vi "canDataSort.vi"() -> ()   [LabVIEW 2023] (continued)
1072  1FFFFFFF   00000004    8        00\t20\tFF\tFF\tFF\tFF\tFF\tFF\r\n      1063  0CF102A7   00000004    8        30\t75\tE0\t2E\t80\tFF\tFF\tFD\r\n      1063  0CF101A7   00000004    8        68\t00\t97\tCC\t00\t15\t39\t4F\r\n      1062  1FFFFFFF   00000004    8        00\t20\tFF\tFF\tFF\tFF\tFF\tFF\r\n      1052  1FFFFFFF   00000004    8        00\t00\tFF\tFF\tFF\tFF\tFF\tFF\r\n      1047  1FFFFFFF   00000004    8        00\t00\tFF\tFF\tFF\tFF\tFF\tFF\r\n      1046  18F121F0   00000004    8        09\t18\t00\t00\tFF\tFF\tB0\t01\r\n      1045  18F106A7   00000004    8        00\tF7\tFF\tFF\tFF\tFF\tFF\t85\r\n      1045  0CF104A7   00000004    8        F0\t60\t22\tFC\tFF\tFF\tFF\t42\r\n      1044  0CF103A7   00000004    8        17\t1F\t08\t60\tB1\t1F\t08\t42\r\n      1044  0CF102A7   00000004    8        30\t75\tE0\t2E\t80\tFF\tFF\tFD\r\n      1082  1FFFFFFF   00000004    8        00\t20\tFF\tFF\tFF\tFF\tFF\tFF\r\n      1072  1FFFFFFF   00000004    8        00\t20\tFF\tFF\tFF\tFF\tFF\tFF\r\n      1063  0CF102A7   00000004    8        30\t75\tE0\t2E\t80\tFF\tFF\tFD\r\n      1063  0CF101A7   00000004    8        68\t00\t97\tCC\t00\t15\t39\t4F\r\n      1062  1FFFFFFF   00000004    8        00\t20\tFF\tFF\tFF\tFF\tFF\tFF\r\n      1052  1FFFFFFF   00000004    8        00\t00\tFF\tFF\tFF\tFF\tFF\tFF\r\n      1047  1FFFFFFF   00000004    8        00\t00\tFF\tFF\tFF\tFF\tFF\tFF\r\n      1046  18F121F0   00000004    8        09\t18\t00\t00\tFF\tFF\tB0\t01\r\n      1045  18F106A7   00000004    8        00\tF7\tFF\tFF\tFF\tFF\tFF\t85\r\n      1045  0CF104A7   00000004    8        F0\t60\t22\tFC\tFF\tFF\tFF\t42\r\n      1044  0CF103A7   00000004    8        17\t1F\t08\t60\tB1\t1F\t08\t42\r\n      1083  0CF101A7   00000004    8        68\t00\t97\tCC\t00\t15\t39\t50\r\n      1082  1FFFFFFF   00000004    8        00\t20\tFF\tFF\tFF\tFF\tFF\tFF\r\n      1072  1FFFFFFF   00000004    8        00\t20\tFF\tFF\tFF\tFF\tFF\tFF\r\n      1063  0CF102A7   00000004    8        30\t75\tE0\t2E\t80\tFF\tFF\tFD\r\n      1063  0CF101A7   00000004    8        68\t00\t97\tCC\t00\t15\t39\t4F\r\n      1062  1FFFFFFF   00000004    8        00\t20\tFF\tFF\tFF\tFF\tFF\tFF\r\n      1052  1FFFFFFF   00000004    8        00\t00\tFF\tFF\tFF\tFF\tFF\tFF\r\n      1047  1FFFFFFF   00000004    8        00\t00\tFF\tFF\tFF\tFF\tFF\tFF\r\n      1046  18F121F0   00000004    8        09\t18\t00\t00\tFF\tFF\tB0\t01\r\n      1045  18F106A7   00000004    8        00\tF7\tFF\tFF\tFF\tFF\tFF\t85\r\n      1045  0CF104A7   00000004    8        F0\t60\t22\tFC\tFF\tFF\tFF\t42\r\n      1083  0CF102A7   00000004    8        30\t75\tE0\t2E\t80\tFF\tFF\tFD\r\n      1083  0CF101A7   00000004    8        68\t00\t97\tCC\t00\t15\t39\t50\r\n      1082  1FFFFFFF   00000004    8        00\t20\tFF\tFF\tFF\tFF\tFF\tFF\r\n      1072  1FFFFFFF   00000004    8        00\t20\tFF\tFF\tFF\tFF\tFF\tFF\r\n      1063  0CF102A7   00000004    8        30\t75\tE0\t2E\t80\tFF\tFF\tFD\r\n      1063  0CF101A7   00000004    8        68\t00\t97\tCC\t00\t15\t39\t4F\r\n      1062  1FFFFFFF   00000004    8        00\t20\tFF\tFF\tFF\tFF\tFF\tFF\r\n      1052  1FFFFFFF   00000004    8        00\t00\tFF\tFF\tFF\tFF\tFF\tFF\r\n      1047  1FFFFFFF   00000004    8        00\t00\tFF\tFF\tFF\tFF\tFF\tFF\r\n      1046  18F121F0   00000004    8        09\t18\t00\t00\tFF\tFF\tB0\t01\r\n      1045  18F106A7   00000004    8        00\tF7\tFF\tFF\tFF\tFF\tFF\t85\r\n      1092  1FFFFFFF   00000004    8        00\t00\tFF\tFF\tFF\tFF\tFF\tFF\r\n      1083  0CF102A7   00000004    8        30\t75\tE0\t2E\t80\tFF\tFF\tFD\r\n      1083  0CF101A7   00000004    8        68\t00\t97\tCC\t00\t15\t39\t50\r\n      1082  1FFFFFFF   00000004    8        00\t20\tFF\tFF\tFF\tFF\tFF\tFF\r\n      1072  1FFFFFFF   00000004    8        00\t20\tFF\tFF\tFF\tFF\tFF\tFF\r\n      1063  0CF102A7   00000004    8        30\t75\tE0\t2E\t80\tFF\tFF\tFD\r\n      1063  0CF101A7   00000004    8        68\t00\t97\tCC\t00\t15\t39\t4F\r\n      1062  1FFFFFFF   00000004    8        00\t20\tFF\tFF\tFF\tFF\tFF\tFF\r\n      1052  1FFFFFFF   00000004    8        00\t00\tFF\tFF\tFF\tFF\tFF\tFF\r\n      1047  1FFFFFFF   00000004    8        00\t00\tFF\tFF\tFF\tFF\tFF\tFF\r\n      1046  18F121F0   00000004    8        09\t18\t00\t00\tFF\tFF\tB0\t01\r\n      1093  18F106A7   00000004    8        00\tF7\tFF\tFF\tFF\tFF\tFF\t86\r\n      1092  1FFFFFFF   00000004    8        00\t00\tFF\tFF\tFF\tFF\tFF\tFF\r\n      1083  0CF102A7   00000004    8        30\t75\tE0\t2E\t80\tFF\tFF\tFD\r\n      1083  0CF101A7   00000004    8        68\t00\t97\tCC\t00\t15\t39\t50\r\n      1082  1FFFFFFF   00000004    8        00\t20\tFF\tFF\tFF\tFF\tFF\tFF\r\n      1072  1FFFFFFF   00000004    8        00\t20\tFF\tFF\tFF\tFF\tFF\tFF\r\n      1063  0CF102A7   00000004    8        30\t75\tE0\t2E\t80\tFF\tFF\tFD\r\n      1063  0CF101A7   00000004    8        68\t00\t97\tCC\t00\t15\t39\t4F\r\n      1062  1FFFFFFF   00000004    8        00\t20\tFF\tFF\tFF\tFF\tFF\tFF\r\n      1052  1FFFFFFF   00000004    8        00\t00\tFF\tFF\tFF\tFF\tFF\tFF\r\n      1047  1FFFFFFF   00000004    8        00\t00\tFF\tFF\tFF\tFF\tFF\tFF\r\n      1102  1FFFFFFF   00000004    8        00\t20\tFF\tFF\tFF\tFF\tFF\tFF\r\n      1093  18F106A7   00000004    8        00\tF7\tFF\tFF\tFF\tFF\tFF\t86\r\n      1092  1FFFFFFF   00000004    8        00\t00\tFF\tFF\tFF\tFF\tFF\tFF\r\n      1083  0CF102A7   00000004    8        30\t75\tE0\t2E\t80\tFF\tFF\tFD\r\n      1083  0CF101A7   00000004    8        68\t00\t97\tCC\t00\t15\t39\t50\r\n      1082  1FFFFFFF   00000004    8        00\t20\tFF\tFF\tFF\tFF\tFF\tFF\r\n      1072  1FFFFFFF   00000004    8        00\t20\tFF\tFF\tFF\tFF\tFF\tFF\r\n      1063  0CF102A7   00000004    8        30\t75\tE0\t2E\t80\tFF\tFF\tFD\r\n      1063  0CF101A7   00000004    8        68\t00\t97\tCC\t00\t15\t39\t4F\r\n      1062  1FFFFFFF   00000004    8        00\t20\tFF\tFF\tFF\tFF\tFF\tFF\r\n      1052  1FFFFFFF   00000004    8        00\t00\tFF\tFF\tFF\tFF\tFF\tFF\r\n      1103  0CF101A7   00000004    8        68\t00\t97\tCC\t00\t15\t39\t51\r\n      1102  1FFFFFFF   00000004    8        00\t20\tFF\tFF\tFF\tFF\tFF\tFF\r\n      1093  18F106A7   00000004    8        00\tF7\tFF\tFF\tFF\tFF\tFF\t86\r\n      1092  1FFFFFFF   00000004    8        00\t00\tFF\tFF\tFF\tFF\tFF\tFF\r\n      1083  0CF102A7   00000004    8        30\t75\tE0\t2E\t80\tFF\tFF\tFD\r\n      1083  0CF101A7   00000004    8        68\t00\t97\tCC\t00\t15\t39\t50\r\n      1082  1FFFFFFF   00000004    8        00\t20\tFF\tFF\tFF\tFF\tFF\tFF\r\n      1072  1FFFFFFF   00000004    8        00\t20\tFF\tFF\tFF\tFF\tFF\tFF\r\n      1063  0CF102A7   00000004    8        30\t75\tE0\t2E\t80\tFF\tFF\tFD\r\n      1063  0CF101A7   00000004    8        68\t00\t97\tCC\t00\t15\t39\t4F\r\n      1062  1FFFFFFF   00000004    8        00\t20\tFF\tFF\tFF\tFF\tFF\tFF\r\n      1103  0CF102A7   00000004    8        30\t75\tE0\t2E\t80\tFF\tFF\tFD\r\n      1103  0CF101A7   00000004    8        68\t00\t97\tCC\t00\t15\t39\t51\r\n      1102  1FFFFFFF   00000004    8        00\t20\tFF\tFF\tFF\tFF\tFF\tFF\r\n      1093  18F106A7   00000004    8        00\tF7\tFF\tFF\tFF\tFF\tFF\t86\r\n      1092  1FFFFFFF   00000004    8        00\t00\tFF\tFF\tFF\tFF\tFF\tFF\r\n      1083  0CF102A7   00000004    8        30\t75\tE0\t2E\t80\tFF\tFF\tFD\r\n      1083  0CF101A7   00000004    8        68\t00\t97\tCC\t00\t15\t39\t50\r\n      1082  1FFFFFFF   00000004    8        00\t20\tFF\tFF\tFF\tFF\tFF\tFF\r\n      1072  1FFFFFFF   00000004    8        00\t20\tFF\tFF\tFF\tFF\tFF\tFF\r\n      1063  0CF102A7   00000004    8        30\t75\tE0\t2E\t80\tFF\tFF\tFD\r\n      1063  0CF101A7   00000004    8        68\t00\t97\tCC\t00\t15\t39\t4F\r\n      1112  1FFFFFFF   00000004    8        00\t20\tFF\tFF\tFF\tFF\tFF\tFF\r\n      1103  0CF102A7   00000004    8        30\t75\tE0\t2E\t80\tFF\tFF\tFD\r\n      1103  0CF101A7   00000004    8        68\t00\t97\tCC\t00\t15\t39\t51\r\n      1102  1FFFFFFF   00000004    8        00\t20\tFF\tFF\tFF\tFF\tFF\tFF\r\n      1093  18F106A7   00000004    8        00\tF7\tFF\tFF\tFF\tFF\tFF\t86\r\n      1092  1FFFFFFF   00000004    8        00\t00\tFF\tFF\tFF\tFF\tFF\tFF\r\n      1083  0CF102A7   00000004    8        30\t75\tE0\t2E\t80\tFF\tFF\tFD\r\n      1083  0CF101A7   00000004    8        68\t00\t97\tCC\t00\t15\t39\t50\r\n      1082  1FFFFFFF   00000004    8        00\t20\tFF\tFF\tFF\tFF\tFF\tFF\r\n      1072  1FFFFFFF   00000004    8        00\t20\tFF\tFF\tFF\tFF\tFF\tFF\r\n      1063  0CF102A7   00000004    8        30\t75\tE0\t2E\t80\tFF\tFF\tFD\r\n      1122  1FFFFFFF   00000004    8        00\t20\tFF\tFF\tFF\tFF\tFF\tFF\r\n      1112  1FFFFFFF   00000004    8        00\t20\tFF\tFF\tFF\tFF\tFF\tFF\r\n      1103  0CF102A7   00000004    8        30\t75\tE0\t2E\t80\tFF\tFF\tFD\r\n      1103  0CF101A7   00000004    8        68\t00\t97\tCC\t00\t15\t39\t51\r\n      1102  1FFFFFFF   00000004    8        00\t20\tFF\tFF\tFF\tFF\tFF\tFF\r\n      1093  18F106A7   00000004    8        00\tF7\tFF\tFF\tFF\tFF\tFF\t86\r\n      1092  1FFFFFFF   00000004    8        00\t00\tFF\tFF\tFF\tFF\tFF\tFF\r\n      1083  0CF102A7   00000004    8        30\t75\tE0\t2E\t80\tFF\tFF\tFD\r\n      1083  0CF101A7   00000004    8        68\t00\t97\tCC\t00\t15\t39\t50\r\n      1082  1FFFFFFF   00000004    8        00\t20\tFF\tFF\tFF\tFF\tFF\tFF\r\n      1072  1FFFFFFF   00000004    8        00\t20\tFF\tFF\tFF\tFF\tFF\tFF\r\n      1123  0CF101A7   00000004    8        68\t00\t97\tCC\t00\t15\t39\t52\r\n      1122  1FFFFFFF   00000004    8        00\t20\tFF\tFF\tFF\tFF\tFF\tFF\r\n      1112  1FFFFFFF   00000004    8        00\t20\tFF\tFF\tFF\tFF\tFF\tFF\r\n      1103  0CF102A7   00000004    8        30\t75\tE0\t2E\t80\tFF\tFF\tFD\r\n      1103  0CF101A7   00000004    8        68\t00\t97\tCC\t00\t15\t39\t51\r\n      1102  1FFFFFFF   00000004    8        00\t20\tFF\tFF\tFF\tFF\tFF\tFF\r\n      1093  18F106A7   00000004    8        00\tF7\tFF\tFF\tFF\tFF\tFF\t86\r\n      1092  1FFFFFFF   00000004    8        00\t00\tFF\tFF\tFF\tFF\tFF\tFF\r\n      1083  0CF102A7   00000004    8        30\t75\tE0\t2E\t80\tFF\tFF\tFD\r\n      1083  0CF101A7   00000004    8        68\t00\t97\tCC\t00\t15\t39\t50\r\n      1082  1FFFFFFF   00000004    8        00\t20\tFF\tFF\tFF\tFF\tFF\tFF\r\n      1123  0CF102A7   00000004    8        30\t75\tE0\t2E\t80\tFF\tFF\tFD\r\n      1123  0CF101A7   00000004    8        68\t00\t97\tCC\t00\t15\t39\t52\r\n      1122  1FFFFFFF   00000004    8        00\t20\tFF\tFF\tFF\tFF\tFF\tFF\r\n      1112  1FFFFFFF   00000004    8        00\t20\tFF\tFF\tFF\tFF\tFF\tFF\r\n      1103  0CF102A7   00000004    8        30\t75\tE0\t2E\t80\tFF\tFF\tFD\r\n      1103  0CF101A7   00000004    8        68\t00\t97\tCC\t00\t15\t39\t51\r\n      1102  1FFFFFFF   00000004    8        00\t20\tFF\tFF\tFF\tFF\tFF\tFF\r\n      1093  18F106A7   00000004    8        00\tF7\tFF\tFF\tFF\tFF\tFF\t86\r\n      1092  1FFFFFFF   00000004    8        00\t00\tFF\tFF\tFF\tFF\tFF\tFF\r\n      1083  0CF102A7   00000004    8        30\t75\tE0\t2E\t80\tFF\tFF\tFD\r\n      1083  0CF101A7   00000004    8        68\t00\t97\tCC\t00\t15\t39\t50\r\n      1132  1FFFFFFF   00000004    8        00\t20\tFF\tFF\tFF\tFF\tFF\tFF\r\n      1123  0CF102A7   00000004    8        30\t75\tE0\t2E\t80\tFF\tFF\tFD\r\n      1123  0CF101A7   00000004    8        68\t00\t97\tCC\t00\t15\t39\t52\r\n      1122  1FFFFFFF   00000004    8        00\t20\tFF\tFF\tFF\tFF\tFF\tFF\r\n      1112  1FFFFFFF   00000004    8        00\t20\tFF\tFF\tFF\tFF\tFF\tFF\r\n      1103  0CF102A7   00000004    8        30\t75\tE0\t2E\t80\tFF\tFF\tFD\r\n      1103  0CF101A7   00000004    8        68\t00\t97\tCC\t00\t15\t39\t51\r\n      1102  1FFFFFFF   00000004    8        00\t20\tFF\tFF\tFF\tFF\tFF\tFF\r\n      1093  18F106A7   00000004    8        00\tF7\tFF\tFF\tFF\tFF\tFF\t86\r\n      1092  1FFFFFFF   00000004    8        00\t00\tFF\tFF\tFF\tFF\tFF\tFF\r\n      1083  0CF102A7   00000004    8        30\t75\tE0\t2E\t80\tFF\tFF\tFD\r\n      1141  18F11FF0   00000004    8        FF\t3F\t90\t68\t88\t1B\t10\t3C\r\n      1132  1FFFFFFF   00000004    8        00\t20\tFF\tFF\tFF\tFF\tFF\tFF\r\n      1123  0CF102A7   00000004    8        30\t75\tE0\t2E\t80\tFF\tFF\tFD\r\n      1123  0CF101A7   00000004    8        68\t00\t97\tCC\t00\t15\t39\t52\r\n      1122  1FFFFFFF   00000004    8        00\t20\tFF\tFF\tFF\tFF\tFF\tFF\r\n      1112  1FFFFFFF   00000004    8        00\t20\tFF\tFF\tFF\tFF\tFF\tFF\r\n      1103  0CF102A7   00000004    8        30\t75\tE0\t2E\t80\tFF\tFF\tFD\r\n      1103  0CF101A7   00000004    8        68\t00\t97\tCC\t00\t15\t39\t51\r\n      1102  1FFFFFFF   00000004    8        00\t20\tFF\tFF\tFF\tFF\tFF\tFF\r\n      1093  18F106A7   00000004    8        00\tF7\tFF\tFF\tFF\tFF\tFF\t86\r\n      1092  1FFFFFFF   00000004    8        00\t00\tFF\tFF\tFF\tFF\tFF\tFF\r\n      1142  18F120F0   00000004    8        2B\t75\t60\tB1\tB0\t01\tFF\tFF\r\n      1141  18F11FF0   00000004    8        FF\t3F\t90\t68\t88\t1B\t10\t3C\r\n      1132  1FFFFFFF   00000004    8        00\t20\tFF\tFF\tFF\tFF\tFF\tFF\r\n      1123  0CF102A7   00000004    8        30\t75\tE0\t2E\t80\tFF\tFF\tFD\r\n      1123  0CF101A7   00000004    8        68\t00\t97\tCC\t00\t15\t39\t52\r\n      1122  1FFFFFFF   00000004    8        00\t20\tFF\tFF\tFF\tFF\tFF\tFF\r\n      1112  1FFFFFFF   00000004    8        00\t20\tFF\tFF\tFF\tFF\tFF\tFF\r\n      1103  0CF102A7   00000004    8        30\t75\tE0\t2E\t80\tFF\tFF\tFD\r\n      1103  0CF101A7   00000004    8        68\t00\t97\tCC\t00\t15\t39\t51\r\n      1102  1FFFFFFF   00000004    8        00\t20\tFF\tFF\tFF\tFF\tFF\tFF\r\n      1093  18F106A7   00000004    8        00\tF7\tFF\tFF\tFF\tFF\tFF\t86\r\n      1143  0CF101A7   00000004    8        68\t00\t97\tCC\t00\t15\t39\t53\r\n      1142  18F120F0   00000004    8        2B\t75\t60\tB1\tB0\t01\tFF\tFF\r\n      1141  18F11FF0   00000004    8        FF\t3F\t90\t68\t88\t1B\t10\t3C\r\n      1132  1FFFFFFF   00000004    8        00\t20\tFF\tFF\tFF\tFF\tFF\tFF\r\n      1123  0CF102A7   00000004    8        30\t75\tE0\t2E\t80\tFF\tFF\tFD\r\n      1123  0CF101A7   00000004    8        68\t00\t97\tCC\t00\t15\t39\t52\r\n      1122  1FFFFFFF   00000004    8        00\t20\tFF\tFF\tFF\tFF\tFF\tFF\r\n      1112  1FFFFFFF   00000004    8        00\t20\tFF\tFF\tFF\tFF\tFF\tFF\r\n      1103  0CF102A7   00000004    8        30\t75\tE0\t2E\t80\tFF\tFF\tFD\r\n      1103  0CF101A7   00000004    8        68\t00\t97\tCC\t00\t15\t39\t51\r\n      1102  1FFFFFFF   00000004    8        00\t20\tFF\tFF\tFF\tFF\tFF\tFF\r\n      1143  0C3C4D4A   00000004    8        BE\tFF\tFF\t7F\t18\tFF\tFF\t43\r\n      1143  0CF101A7   00000004    8        68\t00\t97\tCC\t00\t15\t39\t53\r\n      1142  18F120F0   00000004    8        2B\t75\t60\tB1\tB0\t01\tFF\tFF\r\n      1141  18F11FF0   00000004    8        FF\t3F\t90\t68\t88\t1B\t10\t3C\r\n      1132  1FFFFFFF   00000004    8        00\t20\tFF\tFF\tFF\tFF\tFF\tFF\r\n      1123  0CF102A7   00000004    8        30\t75\tE0\t2E\t80\tFF\tFF\tFD\r\n      1123  0CF101A7   00000004    8        68\t00\t97\tCC\t00\t15\t39\t52\r\n      1122  1FFFFFFF   00000004    8        00\t20\tFF\tFF\tFF\tFF\tFF\tFF\r\n      1112  1FFFFFFF   00000004    8        00\t20\tFF\tFF\tFF\tFF\tFF\tFF\r\n      1103  0CF102A7   00000004    8        30\t75\tE0\t2E\t80\tFF\tFF\tFD\r\n      1103  0CF101A7   00000004    8        68\t00\t97\tCC\t00\t15\t39\t51\r\n      1144  0CF102A7   00000004    8        30\t75\tE0\t2E\t80\tFF\tFF\tFD\r\n      1143  0C3C4D4A   00000004    8        BE\tFF\tFF\t7F\t18\tFF\tFF\t43\r\n      1143  0CF101A7   00000004    8        68\t00\t97\tCC\t00\t15\t39\t53\r\n      1142  18F120F0   00000004    8        2B\t75\t60\tB1\tB0\t01\tFF\tFF\r\n      1141  18F11FF0   00000004    8        FF\t3F\t90\t68\t88\t1B\t10\t3C\r\n      1132  1FFFFFFF   00000004    8        00\t20\tFF\tFF\tFF\tFF\tFF\tFF\r\n      1123  0CF102A7   00000004    8        30\t75\tE0\t2E\t80\tFF\tFF\tFD\r\n      1123  0CF101A7   00000004    8        68\t00\t97\tCC\t00\t15\t39\t52\r\n      1122  1FFFFFFF   00000004    8        00\t20\tFF\tFF\tFF\tFF\tFF\tFF\r\n      1112  1FFFFFFF   00000004    8        00\t20\tFF\tFF\tFF\tFF\tFF\tFF\r\n      1103  0CF102A7   00000004    8        30\t75\tE0\t2E\t80\tFF\tFF\tFD\r\n      1144  0CF103A7   00000004    8        17\t1F\t08\t60\tB1\t1F\t08\t43\r\n      1144  0CF102A7   00000004    8        30\t75\tE0\t2E\t80\tFF\tFF\tFD\r\n      1143  0C3C4D4A   00000004    8        BE\tFF\tFF\t7F\t18\tFF\tFF\t43\r\n      1143  0CF101A7   00000004    8        68\t00\t97\tCC\t00\t15\t39\t53\r\n      1142  18F120F0   00000004    8        2B\t75\t60\tB1\tB0\t01\tFF\tFF\r\n      1141  18F11FF0   00000004    8        FF\t3F\t90\t68\t88\t1B\t10\t3C\r\n      1132  1FFFFFFF   00000004    8        00\t20\tFF\tFF\tFF\tFF\tFF\tFF\r\n      1123  0CF102A7   00000004    8        30\t75\tE0\t2E\t80\tFF\tFF\tFD\r\n      1123  0CF101A7   00000004    8        68\t00\t97\tCC\t00\t15\t39\t52\r\n      1122  1FFFFFFF   00000004    8        00\t20\tFF\tFF\tFF\tFF\tFF\tFF\r\n      1112  1FFFFFFF   00000004    8        00\t20\tFF\tFF\tFF\tFF\tFF\tFF\r\n      1145  0CF104A7   00000004    8        F0\t60\t22\tFC\tFF\tFF\tFF\t43\r\n      1144  0CF103A7   00000004    8        17\t1F\t08\t60\tB1\t1F\t08\t43\r\n      1144  0CF102A7   00000004    8        30\t75\tE0\t2E\t80\tFF\tFF\tFD\r\n      1143  0C3C4D4A   00000004    8        BE\tFF\tFF\t7F\t18\tFF\tFF\t43\r\n      1143  0CF101A7   00000004    8        68\t00\t97\tCC\t00\t15\t39\t53\r\n      1142  18F120F0   00000004    8        2B\t75\t60\tB1\tB0\t01\tFF\tFF\r\n      1141  18F11FF0   00000004    8        FF\t3F\t90\t68\t88\t1B\t10\t3C\r\n      1132  1FFFFFFF   00000004    8        00\t20\tFF\tFF\tFF\tFF\tFF\tFF\r\n      1123  0CF102A7   00000004    8        30\t75\tE0\t2E\t80\tFF\tFF\tFD\r\n      1123  0CF101A7   00000004    8        68\t00\t97\tCC\t00\t15\t39\t52\r\n      1122  1FFFFFFF   00000004    8        00\t20\tFF\tFF\tFF\tFF\tFF\tFF\r\n      1145  18F106A7   00000004    8        00\tF7\tFF\tFF\tFF\tFF\tFF\t87\r\n      1145  0CF104A7   00000004    8        F0\t60\t22\tFC\tFF\tFF\tFF\t43\r\n      1144  0CF103A7   00000004    8        17\t1F\t08\t60\tB1\t1F\t08\t43\r\n      1144  0CF102A7   00000004    8        30\t75\tE0\t2E\t80\tFF\tFF\tFD\r\n      1143  0C3C4D4A   00000004    8        BE\tFF\tFF\t7F\t18\tFF\tFF\t43\r\n      1143  0CF101A7   00000004    8        68\t00\t97\tCC\t00\t15\t39\t53\r\n      1142  18F120F0   00000004    8        2B\t75\t60\tB1\tB0\t01\tFF\tFF\r\n      1141  18F11FF0   00000004    8        FF\t3F\t90\t68\t88\t1B\t10\t3C\r\n      1132  1FFFFFFF   00000004    8        00\t20\tFF\tFF\tFF\tFF\tFF\tFF\r\n      1123  0CF102A7   00000004    8        30\t75\tE0\t2E\t80\tFF\tFF\tFD\r\n      1123  0CF101A7   00000004    8        68\t00\t97\tCC\t00\t15\t39\t52\r\n      1146  18F108A7   00000004    8        F0\t00\t00\tFF\tFF\tFF\tFF\t40\r\n      1145  18F106A7   00000004    8        00\tF7\tFF\tFF\tFF\tFF\tFF\t87\r\n      1145  0CF104A7   00000004    8        F0\t60\t22\tFC\tFF\tFF\tFF\t43\r\n      1144  0CF103A7   00000004    8        17\t1F\t08\t60\tB1\t1F\t08\t43\r\n      1144  0CF102A7   00000004    8        30\t75\tE0\t2E\t80\tFF\tFF\tFD\r\n      1143  0C3C4D4A   00000004    8        BE\tFF\tFF\t7F\t18\tFF\tFF\t43\r\n      1143  0CF101A7   00000004    8        68\t00\t97\tCC\t00\t15\t39\t53\r\n      1142  18F120F0   00000004    8        2B\t75\t60\tB1\tB0\t01\tFF\tFF\r\n      1141  18F11FF0   00000004    8        FF\t3F\t90\t68\t88\t1B\t10\t3C\r\n      1132  1FFFFFFF   00000004    8        00\t20\tFF\tFF\tFF\tFF\tFF\tFF\r\n      1123  0CF102A7   00000004    8        30\t75\tE0\t2E\t80\tFF\tFF\tFD\r\n      1147  18F121F0   00000004    8        09\t18\t00\t00\tFF\tFF\tB0\t01\r\n      1146  18F108A7   00000004    8        F0\t00\t00\tFF\tFF\tFF\tFF\t40\r\n      1145  18F106A7   00000004    8        00\tF7\tFF\tFF\tFF\tFF\tFF\t87\r\n      1145  0CF104A7   00000004    8        F0\t60\t22\tFC\tFF\tFF\tFF\t43\r\n      1144  0CF103A7   00000004    8        17\t1F\t08\t60\tB1\t1F\t08\t43\r\n      1144  0CF102A7   00000004    8        30\t75\tE0\t2E\t80\tFF\tFF\tFD\r\n      1143  0C3C4D4A   00000004    8        BE\tFF\tFF\t7F\t18\tFF\tFF\t43\r\n      1143  0CF101A7   00000004    8        68\t00\t97\tCC\t00\t15\t39\t53\r\n      1142  18F120F0   00000004    8        2B\t75\t60\tB1\tB0\t01\tFF\tFF\r\n      1141  18F11FF0   00000004    8        FF\t3F\t90\t68\t88\t1B\t10\t3C\r\n      1132  1FFFFFFF   00000004    8        00\t20\tFF\tFF\tFF\tFF\tFF\tFF\r\n      1147  18FEF117   00000004    8        F7\t97\tCC\tCF\tFF\tFF\tFF\tFF\r\n      1147  18F121F0   00000004    8        09\t18\t00\t00\tFF\tFF\tB0\t01\r\n      1146  18F108A7   00000004    8        F0\t00\t00\tFF\tFF\tFF\tFF\t40\r\n      1145  18F106A7   00000004    8        00\tF7\tFF\tFF\tFF\tFF\tFF\t87\r\n      1145  0CF104A7   00000004    8        F0\t60\t22\tFC\tFF\tFF\tFF\t43\r\n      1144  0CF103A7   00000004    8        17\t1F\t08\t60\tB1\t1F\t08\t43\r\n      1144  0CF102A7   00000004    8        30\t75\tE0\t2E\t80\tFF\tFF\tFD\r\n      1143  0C3C4D4A   00000004    8        BE\tFF\tFF\t7F\t18\tFF\tFF\t43\r\n      1143  0CF101A7   00000004    8        68\t00\t97\tCC\t00\t15\t39\t53\r\n      1142  18F120F0   00000004    8        2B\t75\t60\tB1\tB0\t01\tFF\tFF\r\n      1141  18F11FF0   00000004    8        FF\t3F\t90\t68\t88\t1B\t10\t3C\r\n      1148  1FFFFFFF   00000004    8        00\t00\tFF\tFF\tFF\tFF\tFF\tFF\r\n      1147  18FEF117   00000004    8        F7\t97\tCC\tCF\tFF\tFF\tFF\tFF\r\n      1147  18F121F0   00000004    8        09\t18\t00\t00\tFF\tFF\tB0\t01\r\n      1146  18F108A7   00000004    8        F0\t00\t00\tFF\tFF\tFF\tFF\t40\r\n      1145  18F106A7   00000004    8        00\tF7\tFF\tFF\tFF\tFF\tFF\t87\r\n      1145  0CF104A7   00000004    8        F0\t60\t22\tFC\tFF\tFF\tFF\t43\r\n      1144  0CF103A7   00000004    8        17\t1F\t08\t60\tB1\t1F\t08\t43\r\n      1144  0CF102A7   00000004    8        30\t75\tE0\t2E\t80\tFF\tFF\tFD\r\n      1143  0C3C4D4A   00000004    8        BE\tFF\tFF\t7F\t18\tFF\tFF\t43\r\n      1143  0CF101A7   00000004    8        68\t00\t97\tCC\t00\t15\t39\t53\r\n      1142  18F120F0   00000004    8        2B\t75\t60\tB1\tB0\t01\tFF\tFF\r\n      1152  1FFFFFFF   00000004    8        00\t20\tFF\tFF\tFF\tFF\tFF\tFF\r\n      1148  1FFFFFFF   00000004    8        00\t00\tFF\tFF\tFF\tFF\tFF\tFF\r\n      1147  18FEF117   00000004    8        F7\t97\tCC\tCF\tFF\tFF\tFF\tFF\r\n      1147  18F121F0   00000004    8        09\t18\t00\t00\tFF\tFF\tB0\t01\r\n      1146  18F108A7   00000004    8        F0\t00\t00\tFF\tFF\tFF\tFF\t40\r\n      1145  18F106A7   00000004    8        00\tF7\tFF\tFF\tFF\tFF\tFF\t87\r\n      1145  0CF104A7   00000004    8        F0\t60\t22\tFC\tFF\tFF\tFF\t43\r\n      1144  0CF103A7   00000004    8        17\t1F\t08\t60\tB1\t1F\t08\t43\r\n      1144  0CF102A7   00000004    8        30\t75\tE0\t2E\t80\tFF\tFF\tFD\r\n      1143  0C3C4D4A   00000004    8        BE\tFF\tFF\t7F\t18\tFF\tFF\t43\r\n      1143  0CF101A7   00000004    8        68\t00\t97\tCC\t00\t15\t39\t53\r\n      1162  1FFFFFFF   00000004    8        00\t20\tFF\tFF\tFF\tFF\tFF\tFF\r\n      1152  1FFFFFFF   00000004    8        00\t20\tFF\tFF\tFF\tFF\tFF\tFF\r\n      1148  1FFFFFFF   00000004    8        00\t00\tFF\tFF\tFF\tFF\tFF\tFF\r\n      1147  18FEF117   00000004    8        F7\t97\tCC\tCF\tFF\tFF\tFF\tFF\r\n      1147  18F121F0   00000004    8        09\t18\t00\t00\tFF\tFF\tB0\t01\r\n      1146  18F108A7   00000004    8        F0\t00\t00\tFF\tFF\tFF\tFF\t40\r\n      1145  18F106A7   00000004    8        00\tF7\tFF\tFF\tFF\tFF\tFF\t87\r\n      1145  0CF104A7   00000004    8        F0\t60\t22\tFC\tFF\tFF\tFF\t43\r\n      1144  0CF103A7   00000004    8        17\t1F\t08\t60\tB1\t1F\t08\t43\r\n      1144  0CF102A7   00000004    8        30\t75\tE0\t2E\t80\tFF\tFF\tFD\r\n      1143  0C3C4D4A   00000004    8        BE\tFF\tFF\t7F\t18\tFF\tFF\t43\r\n      1163  0CF101A7   00000004    8        68\t00\t97\tCC\t00\t15\t39\t54\r\n      1162  1FFFFFFF   00000004    8        00\t20\tFF\tFF\tFF\tFF\tFF\tFF\r\n      1152  1FFFFFFF   00000004    8        00\t20\tFF\tFF\tFF\tFF\tFF\tFF\r\n      1148  1FFFFFFF   00000004    8        00\t00\tFF\tFF\tFF\tFF\tFF\tFF\r\n      1147  18FEF117   00000004    8        F7\t97\tCC\tCF\tFF\tFF\tFF\tFF\r\n      1147  18F121F0   00000004    8        09\t18\t00\t00\tFF\tFF\tB0\t01\r\n      1146  18F108A7   00000004    8        F0\t00\t00\tFF\tFF\tFF\tFF\t40\r\n      1145  18F106A7   00000004    8        00\tF7\tFF\tFF\tFF\tFF\tFF\t87\r\n      1145  0CF104A7   00000004    8        F0\t60\t22\tFC\tFF\tFF\tFF\t43\r\n      1144  0CF103A7   00000004    8        17\t1F\t08\t60\tB1\t1F\t08\t43\r\n      1144  0CF102A7   00000004    8        30\t75\tE0\t2E\t80\tFF\tFF\tFD\r\n      1163  0CF102A7   00000004    8        30\t75\tE0\t2E\t80\tFF\tFF\tFD\r\n      1163  0CF101A7   00000004    8        68\t00\t97\tCC\t00\t15\t39\t54\r\n      1162  1FFFFFFF   00000004    8        00\t20\tFF\tFF\tFF\tFF\tFF\tFF\r\n      1152  1FFFFFFF   00000004    8        00\t20\tFF\tFF\tFF\tFF\tFF\tFF\r\n      1148  1FFFFFFF   00000004    8        00\t00\tFF\tFF\tFF\tFF\tFF\tFF\r\n      1147  18FEF117   00000004    8        F7\t97\tCC\tCF\tFF\tFF\tFF\tFF\r\n      1147  18F121F0   00000004    8        09\t18\t00\t00\tFF\tFF\tB0\t01\r\n      1146  18F108A7   00000004    8        F0\t00\t00\tFF\tFF\tFF\tFF\t40\r\n      1145  18F106A7   00000004    8        00\tF7\tFF\tFF\tFF\tFF\tFF\t87\r\n      1145  0CF104A7   00000004    8        F0\t60\t22\tFC\tFF\tFF\tFF\t43\r\n      1144  0CF103A7   00000004    8        17\t1F\t08\t60\tB1\t1F\t08\t43\r\n      1172  1FFFFFFF   00000004    8        00\t20\tFF\tFF\tFF\tFF\tFF\tFF\r\n      1163  0CF102A7   00000004    8        30\t75\tE0\t2E\t80\tFF\tFF\tFD\r\n      1163  0CF101A7   00000004    8        68\t00\t97\tCC\t00\t15\t39\t54\r\n      1162  1FFFFFFF   00000004    8        00\t20\tFF\tFF\tFF\tFF\tFF\tFF\r\n      1152  1FFFFFFF   00000004    8        00\t20\tFF\tFF\tFF\tFF\tFF\tFF\r\n      1148  1FFFFFFF   00000004    8        00\t00\tFF\tFF\tFF\tFF\tFF\tFF\r\n      1147  18FEF117   00000004    8        F7\t97\tCC\tCF\tFF\tFF\tFF\tFF\r\n      1147  18F121F0   00000004    8        09\t18\t00\t00\tFF\tFF\tB0\t01\r\n      1146  18F108A7   00000004    8        F0\t00\t00\tFF\tFF\tFF\tFF\t40\r\n      1145  18F106A7   00000004    8        00\tF7\tFF\tFF\tFF\tFF\tFF\t87\r\n      1145  0CF104A7   00000004    8        F0\t60\t22\tFC\tFF\tFF\tFF\t43\r\n      1182  1FFFFFFF   00000004    8        00\t00\tFF\tFF\tFF\tFF\tFF\tFF\r\n      1172  1FFFFFFF   00000004    8        00\t20\tFF\tFF\tFF\tFF\tFF\tFF\r\n      1163  0CF102A7   00000004    8        30\t75\tE0\t2E\t80\tFF\tFF\tFD\r\n      1163  0CF101A7   00000004    8        68\t00\t97\tCC\t00\t15\t39\t54\r\n      1162  1FFFFFFF   00000004    8        00\t20\tFF\tFF\tFF\tFF\tFF\tFF\r\n      1152  1FFFFFFF   00000004    8        00\t20\tFF\tFF\tFF\tFF\tFF\tFF\r\n      1148  1FFFFFFF   00000004    8        00\t00\tFF\tFF\tFF\tFF\tFF\tFF\r\n      1147  18FEF117   00000004    8        F7\t97\tCC\tCF\tFF\tFF\tFF\tFF\r\n      1147  18F121F0   00000004    8        09\t18\t00\t00\tFF\tFF\tB0\t01\r\n      1146  18F108A7   00000004    8        F0\t00\t00\tFF\tFF\tFF\tFF\t40\r\n      1145  18F106A7   00000004    8        00\tF7\tFF\tFF\tFF\tFF\tFF\t87\r\n      1183  0CF101A7   00000004    8        68\t00\t97\tCC\t00\t15\t39\t55\r\n      1182  1FFFFFFF   00000004    8        00\t00\tFF\tFF\tFF\tFF\tFF\tFF\r\n      1172  1FFFFFFF   00000004    8        00\t20\tFF\tFF\tFF\tFF\tFF\tFF\r\n      1163  0CF102A7   00000004    8        30\t75\tE0\t2E\t80\tFF\tFF\tFD\r\n      1163  0CF101A7   00000004    8        68\t00\t97\tCC\t00\t15\t39\t54\r\n      1162  1FFFFFFF   00000004    8        00\t20\tFF\tFF\tFF\tFF\tFF\tFF\r\n      1152  1FFFFFFF   00000004    8        00\t20\tFF\tFF\tFF\tFF\tFF\tFF\r\n      1148  1FFFFFFF   00000004    8        00\t00\tFF\tFF\tFF\tFF\tFF\tFF\r\n      1147  18FEF117   00000004    8        F7\t97\tCC\tCF\tFF\tFF\tFF\tFF\r\n      1147  18F121F0   00000004    8        09\t18\t00\t00\tFF\tFF\tB0\t01\r\n      1146  18F108A7   00000004    8        F0\t00\t00\tFF\tFF\tFF\tFF\t40\r\n      1183  0CF102A7   00000004    8        30\t75\tE0\t2E\t80\tFF\tFF\tFD\r\n      1183  0CF101A7   00000004    8        68\t00\t97\tCC\t00\t15\t39\t55\r\n      1182  1FFFFFFF   00000004    8        00\t00\tFF\tFF\tFF\tFF\tFF\tFF\r\n      1172  1FFFFFFF   00000004    8        00\t20\tFF\tFF\tFF\tFF\tFF\tFF\r\n      1163  0CF102A7   00000004    8        30\t75\tE0\t2E\t80\tFF\tFF\tFD\r\n      1163  0CF101A7   00000004    8        68\t00\t97\tCC\t00\t15\t39\t54\r\n      1162  1FFFFFFF   00000004    8        00\t20\tFF\tFF\tFF\tFF\tFF\tFF\r\n      1152  1FFFFFFF   00000004    8        00\t20\tFF\tFF\tFF\tFF\tFF\tFF\r\n      1148  1FFFFFFF   00000004    8        00\t00\tFF\tFF\tFF\tFF\tFF\tFF\r\n      1147  18FEF117   00000004    8        F7\t97\tCC\tCF\tFF\tFF\tFF\tFF\r\n      1147  18F121F0   00000004    8        09\t18\t00\t00\tFF\tFF\tB0\t01\r\n      1192  1FFFFFFF   00000004    8        00\t20\tFF\tFF\tFF\tFF\tFF\tFF\r\n      1183  0CF102A7   00000004    8        30\t75\tE0\t2E\t80\tFF\tFF\tFD\r\n      1183  0CF101A7   00000004    8        68\t00\t97\tCC\t00\t15\t39\t55\r\n      1182  1FFFFFFF   00000004    8        00\t00\tFF\tFF\tFF\tFF\tFF\tFF\r\n      1172  1FFFFFFF   00000004    8        00\t20\tFF\tFF\tFF\tFF\tFF\tFF\r\n      1163  0CF102A7   00000004    8        30\t75\tE0\t2E\t80\tFF\tFF\tFD\r\n      1163  0CF101A7   00000004    8        68\t00\t97\tCC\t00\t15\t39\t54\r\n      1162  1FFFFFFF   00000004    8        00\t20\tFF\tFF\tFF\tFF\tFF\tFF\r\n      1152  1FFFFFFF   00000004    8        00\t20\tFF\tFF\tFF\tFF\tFF\tFF\r\n      1148  1FFFFFFF   00000004    8        00\t00\tFF\tFF\tFF\tFF\tFF\tFF\r\n      1147  18FEF117   00000004    8        F7\t97\tCC\tCF\tFF\tFF\tFF\tFF\r\n      1193  18F106A7   00000004    8        00\tF7\tFF\tFF\tFF\tFF\tFF\t88\r\n      1192  1FFFFFFF   00000004    8        00\t20\tFF\tFF\tFF\tFF\tFF\tFF\r\n      1183  0CF102A7   00000004    8        30\t75\tE0\t2E\t80\tFF\tFF\tFD\r\n      1183  0CF101A7   00000004    8        68\t00\t97\tCC\t00\t15\t39\t55\r\n      1182  1FFFFFFF   00000004    8        00\t00\tFF\tFF\tFF\tFF\tFF\tFF\r\n      1172  1FFFFFFF   00000004    8        00\t20\tFF\tFF\tFF\tFF\tFF\tFF\r\n      1163  0CF102A7   00000004    8        30\t75\tE0\t2E\t80\tFF\tFF\tFD\r\n      1163  0CF101A7   00000004    8        68\t00\t97\tCC\t00\t15\t39\t54\r\n      1162  1FFFFFFF   00000004    8        00\t20\tFF\tFF\tFF\tFF\tFF\tFF\r\n      1152  1FFFFFFF   00000004    8        00\t20\tFF\tFF\tFF\tFF\tFF\tFF\r\n      1148  1FFFFFFF   00000004    8        00\t00\tFF\tFF\tFF\tFF\tFF\tFF\r\n      1202  1FFFFFFF   00000004    8        00\t00\tFF\tFF\tFF\tFF\tFF\tFF\r\n      1193  18F106A7   00000004    8        00\tF7\tFF\tFF\tFF\tFF\tFF\t88\r\n      1192  1FFFFFFF   00000004    8        00\t20\tFF\tFF\tFF\tFF\tFF\tFF\r\n      1183  0CF102A7   00000004    8        30\t75\tE0\t2E\t80\tFF\tFF\tFD\r\n      1183  0CF101A7   00000004    8        68\t00\t97\tCC\t00\t15\t39\t55\r\n      1182  1FFFFFFF   00000004    8        00\t00\tFF\tFF\tFF\tFF\tFF\tFF\r\n      1172  1FFFFFFF   00000004    8        00\t20\tFF\tFF\tFF\tFF\tFF\tFF\r\n      1163  0CF102A7   00000004    8        30\t75\tE0\t2E\t80\tFF\tFF\tFD\r\n      1163  0CF101A7   00000004    8        68\t00\t97\tCC\t00\t15\t39\t54\r\n      1162  1FFFFFFF   00000004    8        00\t20\tFF\tFF\tFF\tFF\tFF\tFF\r\n      1152  1FFFFFFF   00000004    8        00\t20\tFF\tFF\tFF\tFF\tFF\tFF\r\n      1203  0CF101A7   00000004    8        68\t00\t97\tCC\t00\t15\t39\t56\r\n      1202  1FFFFFFF   00000004    8        00\t00\tFF\tFF\tFF\tFF\tFF\tFF\r\n      1193  18F106A7   00000004    8        00\tF7\tFF\tFF\tFF\tFF\tFF\t88\r\n      1192  1FFFFFFF   00000004    8        00\t20\tFF\tFF\tFF\tFF\tFF\tFF\r\n      1183  0CF102A7   00000004    8        30\t75\tE0\t2E\t80\tFF\tFF\tFD\r\n      1183  0CF101A7   00000004    8        68\t00\t97\tCC\t00\t15\t39\t55\r\n      1182  1FFFFFFF   00000004    8        00\t00\tFF\tFF\tFF\tFF\tFF\tFF\r\n      1172  1FFFFFFF   00000004    8        00\t20\tFF\tFF\tFF\tFF\tFF\tFF\r\n      1163  0CF102A7   00000004    8        30\t75\tE0\t2E\t80\tFF\tFF\tFD\r\n      1163  0CF101A7   00000004    8        68\t00\t97\tCC\t00\t15\t39\t54\r\n      1162  1FFFFFFF   00000004    8        00\t20\tFF\tFF\tFF\tFF\tFF\tFF\r\n      1203  0CF102A7   00000004    8        30\t75\tE0\t2E\t80\tFF\tFF\tFD\r\n      1203  0CF101A7   00000004    8        68\t00\t97\tCC\t00\t15\t39\t56\r\n      1202  1FFFFFFF   00000004    8        00\t00\tFF\tFF\tFF\tFF\tFF\tFF\r\n      1193  18F106A7   00000004    8        00\tF7\tFF\tFF\tFF\tFF\tFF\t88\r\n      1192  1FFFFFFF   00000004    8        00\t20\tFF\tFF\tFF\tFF\tFF\tFF\r\n      1183  0CF102A7   00000004    8        30\t75\tE0\t2E\t80\tFF\tFF\tFD\r\n      1183  0CF101A7   00000004    8        68\t00\t97\tCC\t00\t15\t39\t55\r\n      1182  1FFFFFFF   00000004    8        00\t00\tFF\tFF\tFF\tFF\tFF\tFF\r\n      1172  1FFFFFFF   00000004    8        00\t20\tFF\tFF\tFF\tFF\tFF\tFF\r\n      1163  0CF102A7   00000004    8        30\t75\tE0\t2E\t80\tFF\tFF\tFD\r\n      1163  0CF101A7   00000004    8        68\t00\t97\tCC\t00\t15\t39\t54\r\n      1212  1FFFFFFF   00000004    8        00\t20\tFF\tFF\tFF\tFF\tFF\tFF\r\n      1203  0CF102A7   00000004    8        30\t75\tE0\t2E\t80\tFF\tFF\tFD\r\n      1203  0CF101A7   00000004    8        68\t00\t97\tCC\t00\t15\t39\t56\r\n      1202  1FFFFFFF   00000004    8        00\t00\tFF\tFF\tFF\tFF\tFF\tFF\r\n      1193  18F106A7   00000004    8        00\tF7\tFF\tFF\tFF\tFF\tFF\t88\r\n      1192  1FFFFFFF   00000004    8        00\t20\tFF\tFF\tFF\tFF\tFF\tFF\r\n      1183  0CF102A7   00000004    8        30\t75\tE0\t2E\t80\tFF\tFF\tFD\r\n      1183  0CF101A7   00000004    8        68\t00\t97\tCC\t00\t15\t39\t55\r\n      1182  1FFFFFFF   00000004    8        00\t00\tFF\tFF\tFF\tFF\tFF\tFF\r\n      1172  1FFFFFFF   00000004    8        00\t20\tFF\tFF\tFF\tFF\tFF\tFF\r\n      1163  0CF102A7   00000004    8        30\t75\tE0\t2E\t80\tFF\tFF\tFD\r\n      1222  1FFFFFFF   00000004    8        00\t00\tFF\tFF\tFF\tFF\tFF\tFF\r\n      1212  1FFFFFFF   00000004    8        00\t20\tFF\tFF\tFF\tFF\tFF\tFF\r\n      1203  0CF102A7   00000004    8        30\t75\tE0\t2E\t80\tFF\tFF\tFD\r\n      1203  0CF101A7   00000004    8        68\t00\t97\tCC\t00\t15\t39\t56\r\n      1202  1FFFFFFF   00000004    8        00\t00\tFF\tFF\tFF\tFF\tFF\tFF\r\n      1193  18F106A7   00000004    8        00\tF7\tFF\tFF\tFF\tFF\tFF\t88\r\n      1192  1FFFFFFF   00000004    8        00\t20\tFF\tFF\tFF\tFF\tFF\tFF\r\n      1183  0CF102A7   00000004    8        30\t75\tE0\t2E\t80\tFF\tFF\tFD\r\n      1183  0CF101A7   00000004    8        68\t00\t97\tCC\t00\t15\t39\t55\r\n      1182  1FFFFFFF   00000004    8        00\t00\tFF\tFF\tFF\tFF\tFF\tFF\r\n      1172  1FFFFFFF   00000004    8        00\t20\tFF\tFF\tFF\tFF\tFF\tFF\r\n      1223  0CF101A7   00000004    8        68\t00\t97\tCC\t00\t16\t39\t57\r\n      1222  1FFFFFFF   00000004    8        00\t00\tFF\tFF\tFF\tFF\tFF\tFF\r\n      1212  1FFFFFFF   00000004    8        00\t20\tFF\tFF\tFF\tFF\tFF\tFF\r\n      1203  0CF102A7   00000004    8        30\t75\tE0\t2E\t80\tFF\tFF\tFD\r\n      1203  0CF101A7   00000004    8        68\t00\t97\tCC\t00\t15\t39\t56\r\n      1202  1FFFFFFF   00000004    8        00\t00\tFF\tFF\tFF\tFF\tFF\tFF\r\n      1193  18F106A7   00000004    8        00\tF7\tFF\tFF\tFF\tFF\tFF\t88\r\n      1192  1FFFFFFF   00000004    8        00\t20\tFF\tFF\tFF\tFF\tFF\tFF\r\n      1183  0CF102A7   00000004    8        30\t75\tE0\t2E\t80\tFF\tFF\tFD\r\n      1183  0CF101A7   00000004    8        68\t00\t97\tCC\t00\t15\t39\t55\r\n      1182  1FFFFFFF   00000004    8        00\t00\tFF\tFF\tFF\tFF\tFF\tFF\r\n      1223  0CF102A7   00000004    8        30\t75\tE0\t2E\t80\tFF\tFF\tFD\r\n      1223  0CF101A7   00000004    8        68\t00\t97\tCC\t00\t16\t39\t57\r\n      1222  1FFFFFFF   00000004    8        00\t00\tFF\tFF\tFF\tFF\tFF\tFF\r\n      1212  1FFFFFFF   00000004    8        00\t20\tFF\tFF\tFF\tFF\tFF\tFF\r\n      1203  0CF102A7   00000004    8        30\t75\tE0\t2E\t80\tFF\tFF\tFD\r\n      1203  0CF101A7   00000004    8        68\t00\t97\tCC\t00\t15\t39\t56\r\n      1202  1FFFFFFF   00000004    8        00\t00\tFF\tFF\tFF\tFF\tFF\tFF\r\n      1193  18F106A7   00000004    8        00\tF7\tFF\tFF\tFF\tFF\tFF\t88\r\n      1192  1FFFFFFF   00000004    8        00\t20\tFF\tFF\tFF\tFF\tFF\tFF\r\n      1183  0CF102A7   00000004    8        30\t75\tE0\t2E\t80\tFF\tFF\tFD\r\n      1183  0CF101A7   00000004    8        68\t00\t97\tCC\t00\t15\t39\t55\r\n      1232  1FFFFFFF   00000004    8        00\t20\tFF\tFF\tFF\tFF\tFF\tFF\r\n      1223  0CF102A7   00000004    8        30\t75\tE0\t2E\t80\tFF\tFF\tFD\r\n      1223  0CF101A7   00000004    8        68\t00\t97\tCC\t00\t16\t39\t57\r\n      1222  1FFFFFFF   00000004    8        00\t00\tFF\tFF\tFF\tFF\tFF\tFF\r\n      1212  1FFFFFFF   00000004    8        00\t20\tFF\tFF\tFF\tFF\tFF\tFF\r\n      1203  0CF102A7   00000004    8        30\t75\tE0\t2E\t80\tFF\tFF\tFD\r\n      1203  0CF101A7   00000004    8        68\t00\t97\tCC\t00\t15\t39\t56\r\n      1202  1FFFFFFF   00000004    8        00\t00\tFF\tFF\tFF\tFF\tFF\tFF\r\n      1193  18F106A7   00000004    8        00\tF7\tFF\tFF\tFF\tFF\tFF\t88\r\n      1192  1FFFFFFF   00000004    8        00\t20\tFF\tFF\tFF\tFF\tFF\tFF\r\n      1183  0CF102A7   00000004    8        30\t75\tE0\t2E\t80\tFF\tFF\tFD\r\n      1241  18F11FF0   00000004    8        FF\t3F\t90\t68\t88\t1B\t10\t4C\r\n      1232  1FFFFFFF   00000004    8        00\t20\tFF\tFF\tFF\tFF\tFF\tFF\r\n      1223  0CF102A7   00000004    8        30\t75\tE0\t2E\t80\tFF\tFF\tFD\r\n      1223  0CF101A7   00000004    8        68\t00\t97\tCC\t00\t16\t39\t57\r\n      1222  1FFFFFFF   00000004    8        00\t00\tFF\tFF\tFF\tFF\tFF\tFF\r\n      1212  1FFFFFFF   00000004    8        00\t20\tFF\tFF\tFF\tFF\tFF\tFF\r\n      1203  0CF102A7   00000004    8        30\t75\tE0\t2E\t80\tFF\tFF\tFD\r\n      1203  0CF101A7   00000004    8        68\t00\t97\tCC\t00\t15\t39\t56\r\n      1202  1FFFFFFF   00000004    8        00\t00\tFF\tFF\tFF\tFF\tFF\tFF\r\n      1193  18F106A7   00000004    8        00\tF7\tFF\tFF\tFF\tFF\tFF\t88\r\n      1192  1FFFFFFF   00000004    8        00\t20\tFF\tFF\tFF\tFF\tFF\tFF\r\n      1242  18F120F0   00000004    8        2B\t75\t60\tB1\tB0\t01\tFF\tFF\r\n      1241  18F11FF0   00000004    8        FF\t3F\t90\t68\t88\t1B\t10\t4C\r\n      1232  1FFFFFFF   00000004    8        00\t20\tFF\tFF\tFF\tFF\tFF\tFF\r\n      1223  0CF102A7   00000004    8        30\t75\tE0\t2E\t80\tFF\tFF\tFD\r\n      1223  0CF101A7   00000004    8        68\t00\t97\tCC\t00\t16\t39\t57\r\n      1222  1FFFFFFF   00000004    8        00\t00\tFF\tFF\tFF\tFF\tFF\tFF\r\n      1212  1FFFFFFF   00000004    8        00\t20\tFF\tFF\tFF\tFF\tFF\tFF\r\n      1203  0CF102A7   00000004    8        30\t75\tE0\t2E\t80\tFF\tFF\tFD\r\n      1203  0CF101A7   00000004    8        68\t00\t97\tCC\t00\t15\t39\t56\r\n      1202  1FFFFFFF   00000004    8        00\t00\tFF\tFF\tFF\tFF\tFF\tFF\r\n      1193  18F106A7   00000004    8        00\tF7\tFF\tFF\tFF\tFF\tFF\t88\r\n      1243  0CF101A7   00000004    8        68\t00\t97\tCC\t00\t16\t39\t58\r\n      1242  18F120F0   00000004    8        2B\t75\t60\tB1\tB0\t01\tFF\tFF\r\n      1241  18F11FF0   00000004    8        FF\t3F\t90\t68\t88\t1B\t10\t4C\r\n      1232  1FFFFFFF   00000004    8        00\t20\tFF\tFF\tFF\tFF\tFF\tFF\r\n      1223  0CF102A7   00000004    8        30\t75\tE0\t2E\t80\tFF\tFF\tFD\r\n      1223  0CF101A7   00000004    8        68\t00\t97\tCC\t00\t16\t39\t57\r\n      1222  1FFFFFFF   00000004    8        00\t00\tFF\tFF\tFF\tFF\tFF
